vi "Event Handler.vi"(0 "uService Template in":refnum<class "TCP Listener.lvclass">, 5 "Event type":T1=enum."Message", 7 "Item Name":string, 9 "Data":variant, 11 "error in (no error)":errorcluster) -> (4 "uService Template out":refnum<class "TCP Listener.lvclass">, 15 "error out":errorcluster)   [LabVIEW 2026, in "TALOS.lvlib" / "TCP Listener.lvlib" / "TCP Listener.lvclass"]
uses:
  TCP Listener.lvclass
  C:/LabVIEW Code/TALOS/talos/Father of all uServices/Father of all uServices/Father of all uServices.lvclass
  Father of all uServices/Father of all uServices/Event Handler Items.ctl
  Ancestor/Ancestor/Ancestor.lvclass/Ancestor.ctl
  TCP Listener Consumer Case Selector.ctl
  Father of all uServices/Father of all uServices Messages/Consumer Msg/Consumer Msg.lvclass/Consumer Msg.ctl
  FGV/Error Memory/Get Error Description.vi
  Support VIs/Get PC name.vi
  Ancestor/Ancestor/Read ID.vi
  Support VIs/Get Class Name.vi
  <vilib>/Utility/error.llb/Clear Errors.vi
  Father of all uServices/Father of all uServices Messages/Consumer Msg/Send Consumer.vi
  Support VIs/Substitute Error.vi
  FGV/Error Memory/Error Memory Core.vi
  <vilib>/AdvancedString/Delimited String to 1D String Array.vi
  <vilib>/AdvancedString/Delimited String to 1D String Array (string).vi
  Support VIs/Circus Root Path.vi
  FGV/Error Memory/Error Crt Lvl checker.vi
  FGV/Error Memory/Error Memory Core.vi/40c8088d-b597-4017-91af-faa98e00292e.vi
  FGV/Error Memory/Error Memory Core.vi/d4a3ab98-063c-4e44-b43d-fbdcfe6c2be2.vi
  Father of all uServices/Father of all uServices/Father of all uServices.lvclass
  C:/LabVIEW Code/TALOS/builds/Actor Framework PPL/Actor Framework.lvlibp/1abvi3w/vi.lib/ActorFramework/Actor/Actor.lvclass
  Support VIs/Global Memory.vi
  <vilib>/Utility/LVClass/Get LV Class Name.vi
  Support VIs/Is in Packed Library.vi
  Support VIs/TALOS Root path.vi
  Support VIs/Read CSV worksheet.vi
  Support VIs/Global Constants.vi
  <vilib>/Utility/error.llb/General Error Handler.vi
  builds/Actor Framework PPL/Actor Framework.lvlibp/1abvi3w/vi.lib/ActorFramework/Actor/Read Self Enqueuer.vi
  <userlib>/_OpenG.lib/lvdata/lvdata.llb/Get Strings from Enum__ogtk.vi
  builds/Actor Framework PPL/Actor Framework.lvlibp/1abvi3w/vi.lib/ActorFramework/Message Enqueuer/Enqueue.vi
  Support VIs/Error Log.vi
  Ancestor/Ancestor/Ancestor.lvclass
  <vilib>/Comparison/Equal/Equal Functor/Equal Functor.lvclass
  Father of all uServices/Father of all uServices Messages/Consumer Msg/Consumer Msg.lvclass
  TALOS.lvlib
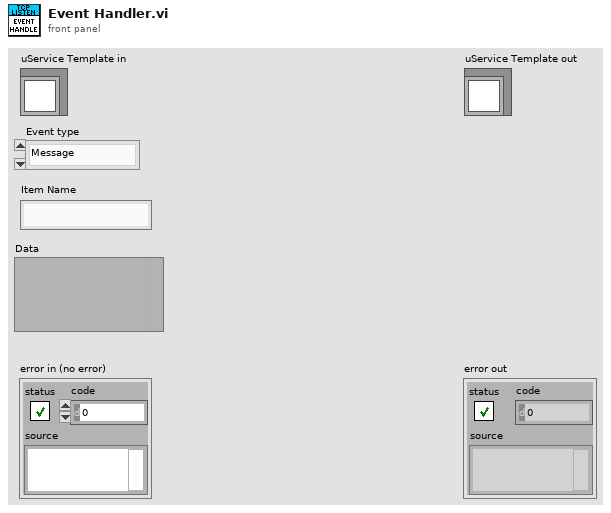
[diagram p1: front panel]
types:
  T1 = typedef "TALOS.lvlib/Father of all uServices.lvlib/Father of all uServices.lvclass/Event Handler Items.ctl" = enum16{"Button Pressed", "Message", "Ready to launch?", "Safe Mode", "Start RUN", "Stop RUN"}
  T2 = typedef "TALOS.lvlib/TCP Listener.lvlib/TCP Listener.lvclass/TCP Listener Consumer Case Selector.ctl" = enum16{"Set Client ID", "Listen", "Idle", "Start accepting connections", "Waiting for connection"}
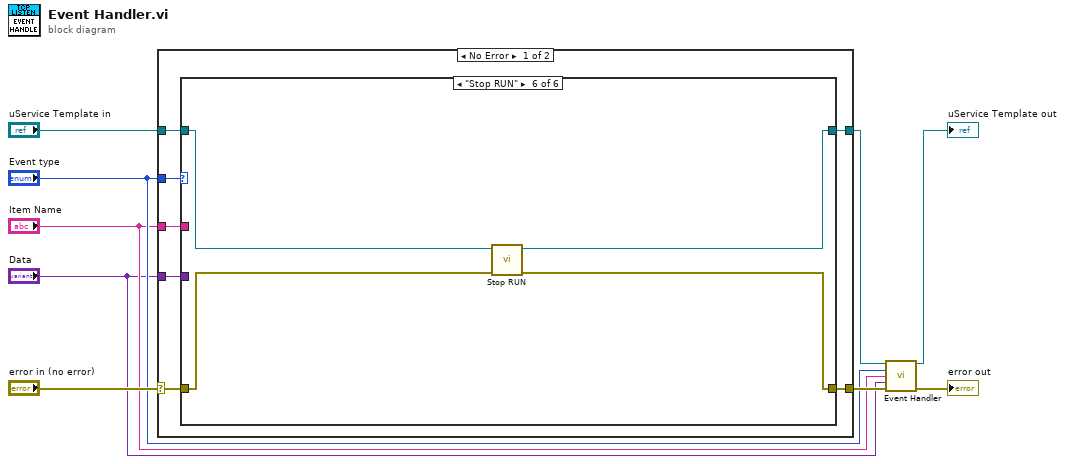
[diagram p0: block diagram]
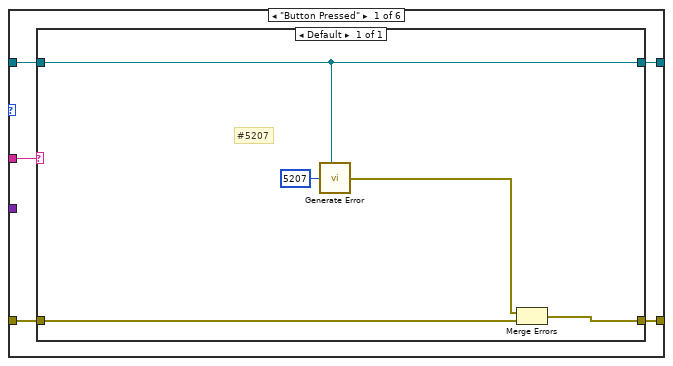
[diagram p2: hidden frame]
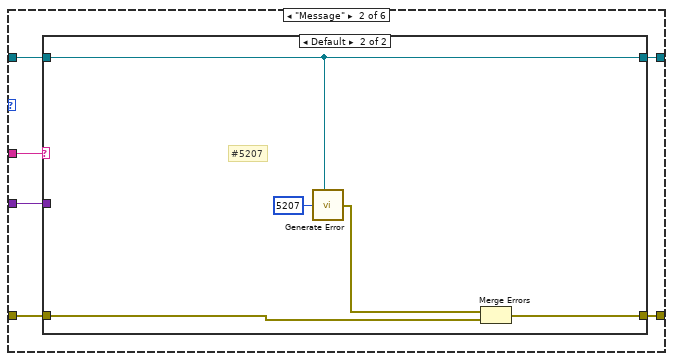
[diagram p3: hidden frame]
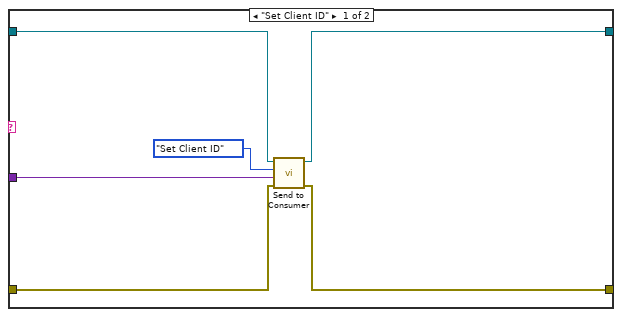
[diagram p4: hidden frame]
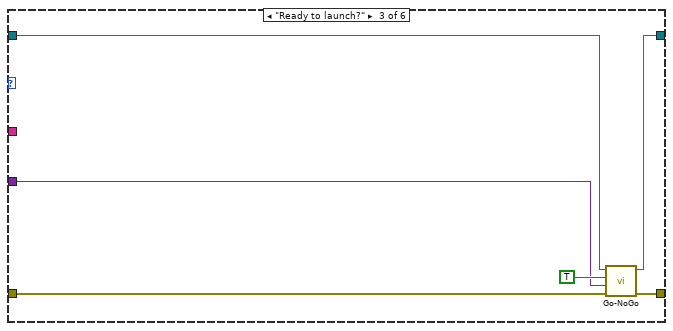
[diagram p5: hidden frame]
diagram:
  n1 = case shown="No Error" "error in (no error)" {
    selector: "error in (no error)" -> [w13 w59]
    tunnel: [w12 w59] -> w7
    tunnel: "uService Template in" -> [w15 w58]
    tunnel: [w14 w58] -> w4
    tunnel: "Event type" -> [w16 _]
    tunnel: "Item Name" -> [w11 _]
    tunnel: "Data" -> [w10 _]
    frame No Error {
      n2 = case shown="\"Stop RUN\"" w16 {
        tunnel: w15 -> [w21 w32 w46 w51 w53 w56]
        tunnel: [w20 w28 w49 w51 w53 w55] -> w14
        tunnel: w13 -> [w17 w29 w47 w50 w52 w57]
        tunnel: [w18 w27 w48 w50 w52 w54] -> w12
        tunnel: w11 -> [w19 w31 _ _ _ _]
        tunnel: w10 -> [_ w30 w44 _ _ _]
        frame "Button Pressed" {
          n3 = case shown="Default" w19 {
            tunnel: w21 -> [w22]
            tunnel: [w22] -> w20
            tunnel: [w25] -> w18
            tunnel: w17 -> [w26]
            frame Default {
              # "#5207"
              n4 = call "Generate Error.vi"("Class"=w22, "Error Code"=5207) -> ("error out"=w24:errorcluster)  [unwired: 5 in]
              n5 = Merge Errors(w24, w26) -> (w25:errorcluster)
            }
          }
        }
        frame "Message" {
          n6 = case shown="Default" w31 {
            tunnel: w32 -> [w38 w41]
            tunnel: w30 -> [w34 _]
            tunnel: w29 -> [w36 w39]
            tunnel: [w37 w41] -> w28
            tunnel: [w35 w40] -> w27
            frame "Set Client ID" {
              n7 = call "Send to Consumer.vi"("error in (no error)"=w36, "Data"=w34, "Case ID"=TCP_Listener_Consumer_Case_Selector."Set Client ID" ("TCP Listener Consumer Case Selector"), "uService Template in"=w38) -> ("error out"=w35:errorcluster, "uService Template out"=w37:refnum<class "TCP Listener.lvclass">)  [unwired: 6 in]
            }
            frame Default {
              # "#5207"
              n8 = call "Generate Error.vi"("Class"=w41, "Error Code"=5207) -> ("error out"=w42:errorcluster)  [unwired: 5 in]
              n9 = Merge Errors(w42, w39) -> (w40:errorcluster)
            }
          }
        }
        frame "Ready to launch?" {
          n10 = call-dynamic "Go-NoGo.vi"("error in (no error)"=w47, "Go-NoGo Data"=w44, "Go?"=TRUE, "Father of all uServices in"=w46) -> ("error out"=w48:errorcluster, "Father of all uServices out"=w49:refnum<class "TCP Listener.lvclass">)  [unwired: 6 in]
        }
        frame "Safe Mode" {
        }
        frame "Start RUN" {
        }
        frame "Stop RUN" {
          n11 = call-dynamic "Stop RUN.vi"("error in (no error)"=w57, "TCP Listener in"=w56) -> ("error out"=w54:errorcluster, "TCP Listener out"=w55:refnum<class "TCP Listener.lvclass">)  [unwired: 8 in]
        }
      }
    }
    frame Error {
    }
  }
  n12 = call-parent "Event Handler.vi"("uService Template in"=w4, "Event type"="Event type", "Item Name"="Item Name", "Data"="Data", "error in (no error)"=w7) -> ("uService Template out"=→"uService Template out":refnum<class "TCP Listener.lvclass">, "error out"=→"error out":errorcluster)  [unwired: 9 in]
